vi "cc_read_temp.vi"(3 "error in (no error)":errorcluster, 4 "Input":u8(ring) items=["A", "B", "C", "D"], 5 "VISA In":refnum<visa-resource-name>) -> (0 "error out":errorcluster, 1 "Temperature":dbl format="%.2f", 2 "VISA Out":refnum<visa-resource-name>)   [LabVIEW 2020]
doc: "Read the current temperature on a selected input."
panel:
  # "Returns numeric\ntemperature reading\nfrom selected input."
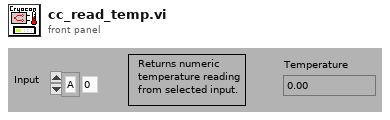
[diagram p1: front panel]
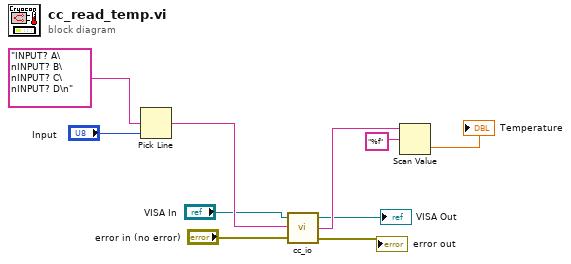
[diagram p0: block diagram]
diagram:
  n1 = Pick Line(multi-line string="INPUT? A\nINPUT? B\nINPUT? C\nINPUT? D\n", line index="Input") -> (output string=w7:string)  [unwired: 1 in]
  n2 = call "cc_io.vi"("error in (no error)"="error in (no error)", "Output Command"=w7, "VISA In"="VISA In") -> ("error out"=→"error out":errorcluster, "Input String"=w4:string, "VISA out"=→"VISA Out":refnum<visa-resource-name>)
  n3 = Scan Value(string=w4, format string="%f") -> (value=→"Temperature":dbl)  [unwired: 1 in, 1 out]
